vi "Sensor Page.vi"(8 "error in (no error)":errorcluster, 11 "Node Ptr":T3 format="%.0x") -> (0 "error out":errorcluster)   [LabVIEW 2018, in "Vires VTD System Explorer.lvlib"]
uses:
  Vires VTD System Explorer.lvlib
  Shared/Protocol.ctl
  Shared/Sensor Name.ctl
  <vilib>/NI Veristand/Custom Device API/Custom Device Item Ref.ctl
  Shared/SensorInfo.ctl
  MM/MM Data.ctl
  MM/MM Objects.ctl
  MM/MM Object.ctl
  <vilib>/NI Veristand/Custom Device API/Get Item Property (Variant).vi
  <vilib>/NI Veristand/Custom Device API/Set Item Property (Variant).vi
  <vilib>/NI Veristand/Custom Device API/Custom Device API.lvlib
  MM/MM.lvlib
  Shared/Vires VTD Shared.lvlib
panel:
  in  "Tab Control":enum32{"Sensor"}(tab)
  in  "PlayerID":u8=1
  in  "# Culled Objects":i32=1
  in  "Network port":i32=48185
  in  "Protocol":T1
  in  "Sensor Name":T2
  in  "SHDocVw.IWebBrowser2":refnum<k7>(container)
  in  "Header":cluster{"Section Name":string}={"Section Name"="Custom Device Item Settings"}
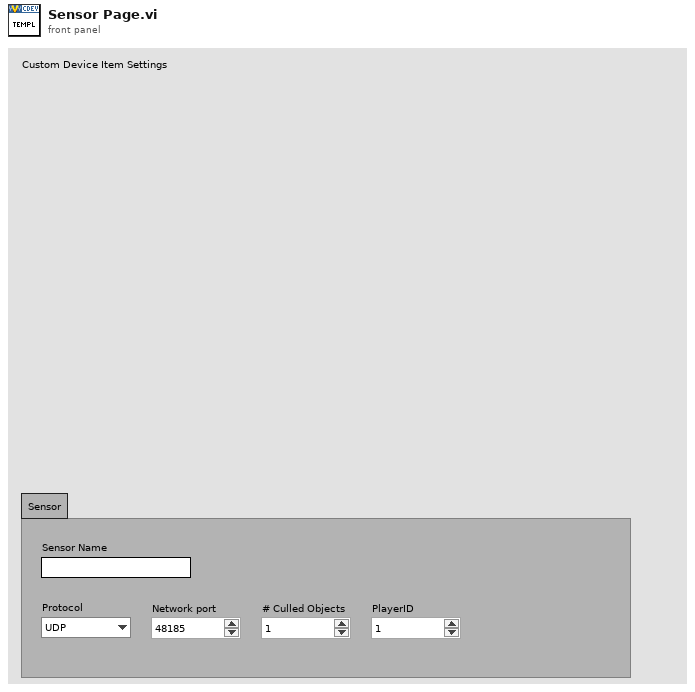
[diagram p1: front panel]
types:
  T1 = typedef "Vires VTD Shared.lvlib/Protocol.ctl" = enum16{"UDP", "TCP"}
  T2 = typedef "Vires VTD Shared.lvlib/Sensor Name.ctl" = string
  T3 = typedef "Custom Device API.lvlib/Custom Device Item Ref.ctl" = u64
  T4 = typedef "Vires VTD Shared.lvlib/SensorInfo.ctl" = cluster{"Sensor Name":T2, "Protocol":T1, "Network port":i32, "# Culled Objects":i32, "PlayerID":u8, "MM Data":T5}
  T5 = typedef "Vires VTD Shared.lvlib/MM Data.ctl" = T6[]
  T6 = typedef "MM.lvlib/MM Objects.ctl" = cluster{"pkID":i32, "MM Objects":T7[]}
  T7 = typedef "MM.lvlib/MM Object.ctl" = cluster{"Object":i32, "Signals":string[]}
  T8 = typedef "Custom Device API.lvlib/Custom Device Commands.ctl" = enum16{"Default", "Item renamed", "Shutdown", "Dynamic button pressed"}
  T9 = typedef "Custom Device API.lvlib/Custom Device Item Info.ctl" = cluster{"Name":string, "Is Channel":bool, "GUID":string, "Is Waveform":bool}
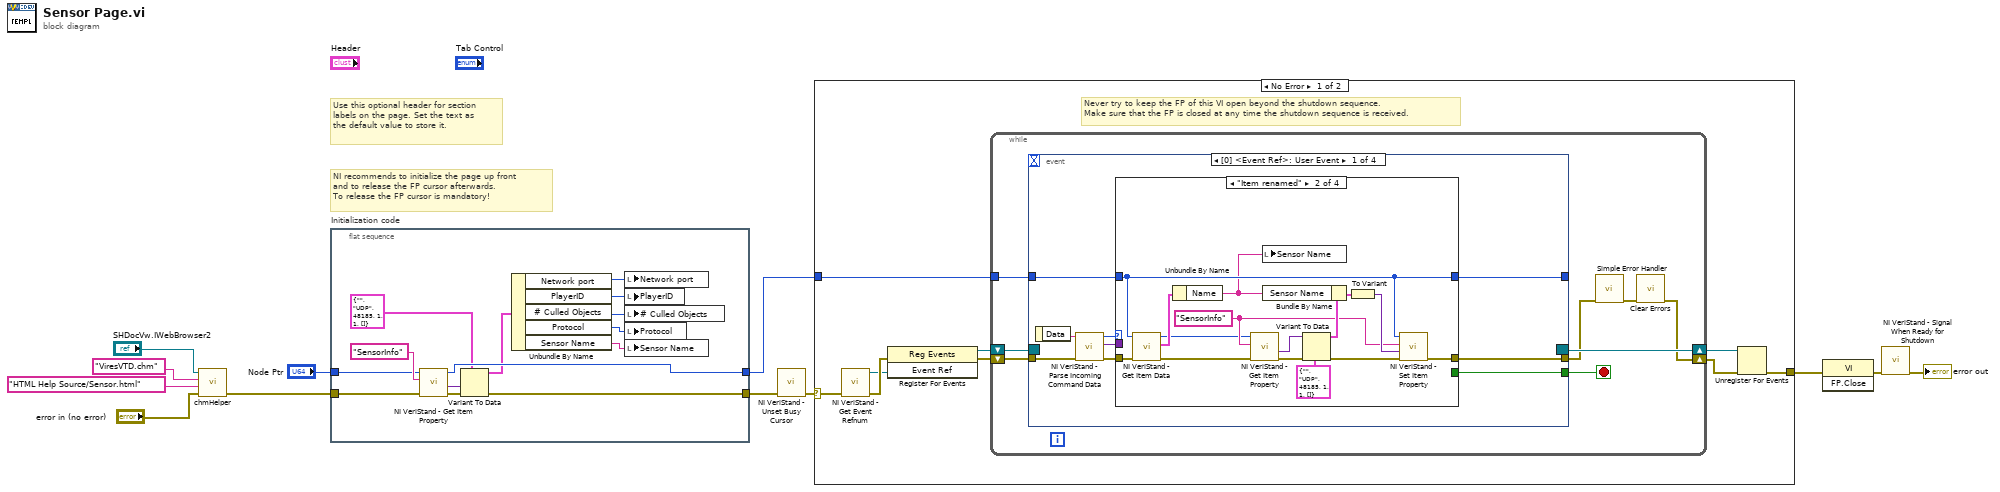
[diagram p0: block diagram]
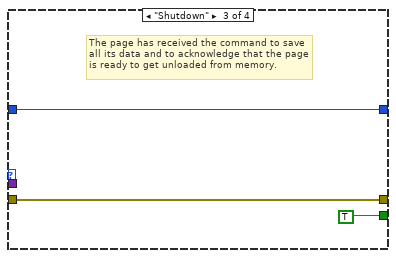
[diagram p3: hidden frame]
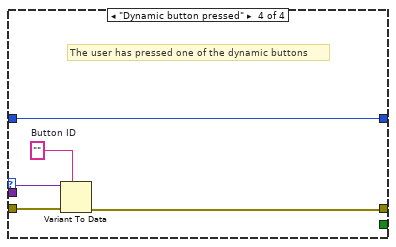
[diagram p4: hidden frame]
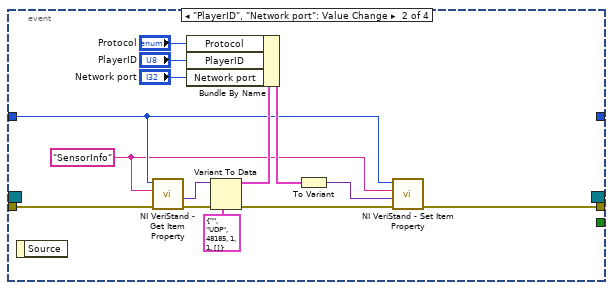
[diagram p5: hidden frame]
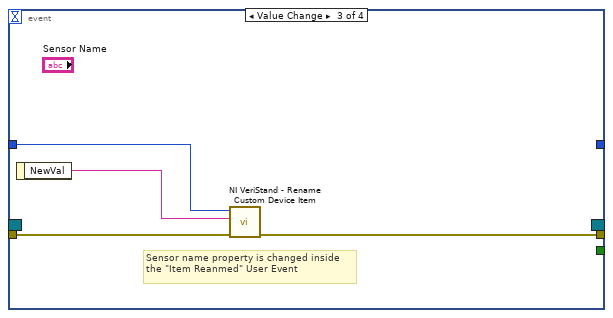
[diagram p6: hidden frame]
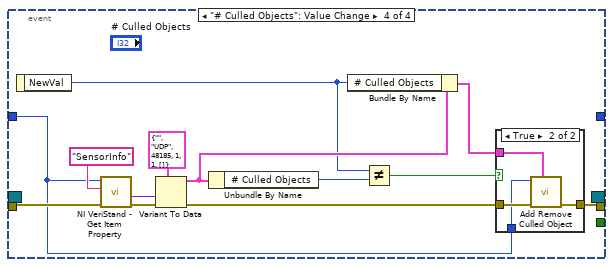
[diagram p7: hidden frame]
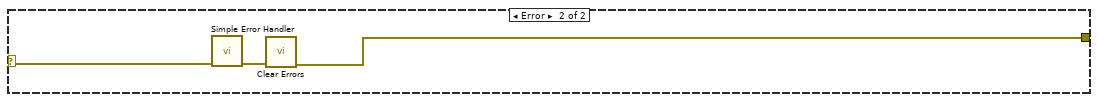
[diagram p9: hidden frame]
diagram:
  # "Use this optional header for section labels on the page. Set the text as the default value to store it."
  # "NI recommends to initialize the page up front\nand to release the FP cursor afterwards.\nTo release the FP cursor is mandatory!"
  n1 = call "chmHelper.vi"("error in (no error)"="error in (no error)", "HTML File"="HTML Help Source/Sensor.html", "Main CHM File"="ViresVTD.chm" ("HTML File"), "Automation Refnum in"="SHDocVw.IWebBrowser2") -> ("error out"=w4:errorcluster)  [unwired: 7 in]
  n2 = flat-sequence "Initialization code" {
    tunnel: w4 -> [w25]
    tunnel: "Node Ptr" -> [w24]
    tunnel: [w21] -> w8
    tunnel: [w23] -> w6
    frame #0 {
      n3 = call-poly <vilib>:"NI VeriStand - Get Item Property.vi"("error in (no error)"=w25, "Property Name"="SensorInfo" ("String"), "Item Ref in"=w24) -> ("error out"=w22:errorcluster, "Value"=w20:variant, "Item Ref out"=w23:T3)  [unwired: 5 in, 1 out]
      n4 = Variant To Data(error in=w22, type=T4 {"Sensor Name"="", "Protocol"=enum."UDP", "Network port"=48185, "# Culled Objects"=1, "PlayerID"=1, "MM Data"=[]} ("SensorInfo"), Variant=w20) -> (data=w18:T4, error out=w21:errorcluster)
      n5 = Unbundle By Name(w18) -> ("Network port"=w17:i32, "PlayerID"=w16:u8, "# Culled Objects"=w15:i32, "Protocol"=w14:T1, "Sensor Name"=w13:T2)
      n6 = local write "Network port"(w17) -> ()
      n7 = local write "PlayerID"(w16) -> ()
      n8 = local write "# Culled Objects"(w15) -> ()
      n9 = local write "Protocol"(w14) -> ()
      n10 = local write "Sensor Name"(w13) -> ()
    }
  }
  n11 = call <vilib>:"NI VeriStand - Unset Busy Cursor.vi"("error in (no error)"=w8) -> ("error out"=w7:errorcluster)  [unwired: 10 out]
  n12 = case shown="No Error" w7 {
    selector: w7 -> [w27 w116]
    tunnel: [w32 w114] -> w12
    tunnel: w6 -> [w28 _]
    frame No Error {
      # "Never try to keep the FP of this VI open beyond the shutdown sequence.\nMake sure that the FP is closed at any time the shutdown sequence is received."
      n13 = call <vilib>:"NI VeriStand - Get Event Refnum.vi"("error in (no error)"=w27) -> ("error out"=w35:errorcluster, "Event Ref"=w31:refnum<user-event>)  [unwired: 9 out]
      n14 = register-events(error in=w35, w31) -> (reference out=w29:refnum<event-registration>, error out=w30:errorcluster)  [unwired: 1 in]
      n15 = while {
        tunnel: w28 -> [w39]
        shift-right: [w36] -> w33
        shift-left: w30 -> [w42]
        shift-right: [w43] -> w34
        shift-left: w29 -> [w41]
        stop <- w40 stop-if-true
        n16 = event shown="[0] <Event Ref>: User Event" {
          selector: w41 -> [_ _ _ _]
          dyn-events: [_ _ _ _] -> w43
          timeout: _ -> [_ _ _ _]
          tunnel: w42 -> [w52 w80 w95 w102]
          tunnel: [w48 _ _ _] -> w40
          tunnel: [w47 w91 w94 w108] -> w38
          tunnel: w39 -> [w46 w79 w92 w97]
          tunnel: [w44 _ _ _] -> _
          event User Event {
            n17 = event-data() -> ("Data"=w51:string)  [unwired: 1 out]
            n18 = call <vilib>:"NI VeriStand - Parse Incoming Command Data.vi"("error in (no error)"=w52, "Incoming data"=w51) -> ("error out"=w50:errorcluster, "Outgoing data"=w45:variant, "Action"=w49:T8)  [unwired: 7 out]
            n19 = case shown="\"Item renamed\"" w49 {
              tunnel: w50 -> [w54 w69 w71 w77]
              tunnel: [_ _ TRUE _] -> w48
              tunnel: [w54 w59 w71 w74] -> w47
              tunnel: w46 -> [w53 w57 w70 w73]
              tunnel: w45 -> [_ _ _ w76]
              tunnel: [w53 w57 w70 w73] -> w44
              frame "Default", Default {
              }
              frame "Item renamed" {
                w58 = "SensorInfo" ("String")
                n20 = call <vilib>:"NI VeriStand - Get Item Data.vi"("error in (no error)"=w69, "Item Ref in"=w57) -> ("error out"=w60:errorcluster, "Item Info"=w68:T9, "Item Ref out"=w56:T3)  [unwired: 7 out]
                n21 = Unbundle By Name(w68) -> ("Name"=w55:string)
                n22 = call-poly <vilib>:"NI VeriStand - Get Item Property.vi"("error in (no error)"=w60, "Property Name"=w58, "Item Ref in"=w56) -> ("error out"=w64:errorcluster, "Value"=w63:variant)  [unwired: 5 in, 2 out]
                n23 = local write "Sensor Name"(w55) -> ()
                n24 = Variant To Data(error in=w64, type=T4 {"Sensor Name"="", "Protocol"=enum."UDP", "Network port"=48185, "# Culled Objects"=1, "PlayerID"=1, "MM Data"=[]} ("SensorInfo"), Variant=w63) -> (data=w62:T4, error out=w67:errorcluster)
                n25 = Bundle By Name(cluster=w62, "Sensor Name"=w55) -> (w66:T4)
                n26 = To Variant(anything=w66) -> (Variant=w65:variant)
                n27 = call-poly <vilib>:"NI VeriStand - Set Item Property.vi"("error in (no error)"=w67, "Value"=w65, "Property Name"=w58, "Item Ref in"=w57) -> ("error out"=w59:errorcluster)  [unwired: 5 in, 2 out]
              }
              frame "Shutdown" {
                # "The page has received the command to save all its data and to acknowledge that the page is ready to get unloaded from memory."
              }
              frame "Dynamic button pressed" {
                w75 = ""  # Button ID
                # "The user has pressed one of the dynamic buttons"
                n28 = Variant To Data(error in=w77, type=w75, Variant=w76) -> (error out=w74:errorcluster)  [unwired: 1 out]
              }
            }
          }
          event "PlayerID", "Network port": Value Change {
            w78 = "SensorInfo" ("String")
            n29 = event-data() -> ()  [unwired: 2 out]
            n30 = call-poly <vilib>:"NI VeriStand - Get Item Property.vi"("error in (no error)"=w80, "Property Name"=w78, "Item Ref in"=w79) -> ("error out"=w85:errorcluster, "Value"=w84:variant)  [unwired: 5 in, 2 out]
            n31 = Variant To Data(error in=w85, type=T4 {"Sensor Name"="", "Protocol"=enum."UDP", "Network port"=48185, "# Culled Objects"=1, "PlayerID"=1, "MM Data"=[]} ("SensorInfo"), Variant=w84) -> (data=w82:T4, error out=w81:errorcluster)
            n32 = Bundle By Name(cluster=w82, "Protocol"="Protocol", "PlayerID"="PlayerID", "Network port"="Network port") -> (w87:T4)
            n33 = To Variant(anything=w87) -> (Variant=w86:variant)
            n34 = call-poly <vilib>:"NI VeriStand - Set Item Property.vi"("error in (no error)"=w81, "Value"=w86, "Property Name"=w78, "Item Ref in"=w79) -> ("error out"=w91:errorcluster)  [unwired: 5 in, 2 out]
          }
          event Value Change {
            # "Sensor name property is changed inside the \"Item Reanmed\" User Event"
            n35 = event-data() -> ("NewVal"=w93:T2)  [unwired: 1 out]
            n36 = call <vilib>:"NI VeriStand - Rename Custom Device Item.vi"("error in (no error)"=w95, "New Name"=w93, "Item Ref in"=w92) -> ("error out"=w94:errorcluster)  [unwired: 6 in, 2 out]
          }
          event "# Culled Objects": Value Change {
            n37 = event-data() -> ("NewVal"=w98:i32)  [unwired: 1 out]
            n38 = call-poly <vilib>:"NI VeriStand - Get Item Property.vi"("error in (no error)"=w102, "Property Name"="SensorInfo" ("String"), "Item Ref in"=w97) -> ("error out"=w106:errorcluster, "Value"=w105:variant)  [unwired: 5 in, 2 out]
            n39 = Variant To Data(error in=w106, type=T4 {"Sensor Name"="", "Protocol"=enum."UDP", "Network port"=48185, "# Culled Objects"=1, "PlayerID"=1, "MM Data"=[]} ("SensorInfo"), Variant=w105) -> (data=w100:T4, error out=w101:errorcluster)
            n40 = Unbundle By Name(w100) -> ("# Culled Objects"=w99:i32)
            n41 = Bundle By Name(cluster=w100, "# Culled Objects"=w98) -> (w107:T4)
            n42 = Not Equal?(x=w98, y=w99) -> (x != y?=w96:bool)
            n43 = case shown="True" w96 {
              tunnel: [w109 w113] -> w108
              tunnel: w107 -> [_ w112]
              tunnel: w101 -> [w109 w111]
              tunnel: w97 -> [_ w110]
              frame False {
              }
              frame True {
                n44 = call "Add Remove Culled Object.vi"("SensorInfo"=w112, "error in (no error)"=w111, "Item Ref in"=w110) -> ("error out (no error)"=w113:errorcluster)  [unwired: 8 in]
              }
            }
          }
        }
        n45 = call <vilib>:"Simple Error Handler.vi"("error in (no error)"=w38) -> ("error out"=w37:errorcluster)  [unwired: 1 in, 7 out]
        n46 = call <vilib>:"Clear Errors.vi"("error in (no error)"=w37) -> ("error out"=w36:errorcluster)  [unwired: 1 in, 5 out]
      }
      n47 = Unregister For Events(event registration refnum=w34, error in=w33) -> (error out=w32:errorcluster)
    }
    frame Error {
      n48 = call <vilib>:"Simple Error Handler.vi"("error in (no error)"=w116) -> ("error out"=w115:errorcluster)  [unwired: 1 in, 7 out]
      n49 = call <vilib>:"Clear Errors.vi"("error in (no error)"=w115) -> ("error out"=w114:errorcluster)  [unwired: 1 in, 5 out]
    }
  }
  n50 = invoke class="VI" method="FP.Close"(error in=w12) -> (error out=w11:errorcluster)  [unwired: 2 in, 2 out]
  n51 = call <vilib>:"NI VeriStand - Signal When Ready for Shutdown.vi"("error in (no error)"=w11) -> ("error out"=→"error out":errorcluster)  [unwired: 10 out]
